vi "Destroy APP UI Display Events.vi"(0 "UI.Event References":T1, 11 "error in":errorcluster) -> (15 "error out":errorcluster)   [LabVIEW 2026, in "Synchronize AWS S3 Content.lvlib"]
doc: "Close user event resources.\n\n<B>Input Parameters</B>\n\n<B>UI display events in</B> references.\n\n<B>error in</B> describes error conditions that occur before this node runs. This input provides standard error in functionality.\n\n<B>Output Parameters</B>\n\n<B>error out</B> contains error information. This output provides standard error out functionality."
uses:
  Synchronize AWS S3 Content.lvlib
  _UI APP Event References.ctl
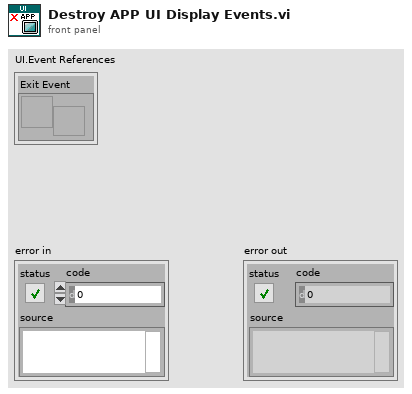
[diagram p1: front panel]
types:
  T1 = typedef "Synchronize AWS S3 Content.lvlib/_UI APP Event References.ctl" = cluster{"Exit Event":refnum<user-event>}
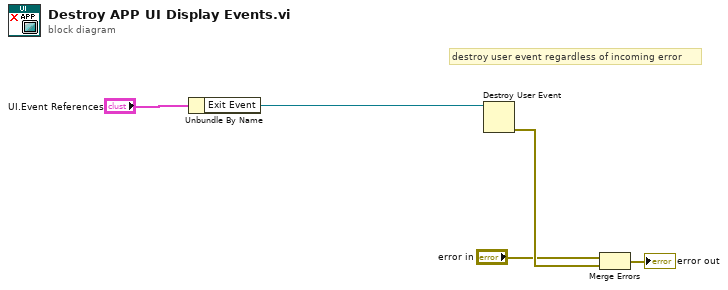
[diagram p0: block diagram]
diagram:
  # "destroy user event regardless of incoming error"
  n1 = Unbundle By Name("UI.Event References") -> ("Exit Event"=w4:refnum<user-event>)
  n2 = Destroy User Event(user event=w4) -> (error out=w3:errorcluster)  [unwired: 1 in]
  n3 = Merge Errors("error in", w3) -> (→"error out":errorcluster)
